vi "ALTS-2015 Write Robot on OPC.vi"(7 "Option":T1=enum."Write Invalid Serial Task", 8 "error in (no error)":errorcluster, 10 "Station # Load":T2, 11 "Serial Details in":T3) -> (0 "error out":errorcluster)   [LabVIEW 2013]
uses:
  Controls/ALTS-2015 Serial Details.ctl
  Controls/ALTS-2015 Station Cluster.ctl
  Controls/ALTS-2015 Write Robot Task OPC Options.ctl
  OPC Engine/Controls/ALTS-2015 OPC Write Global Options.ctl
  OPC Engine/Controls/ALTS-2015 OPC Write Registers.ctl
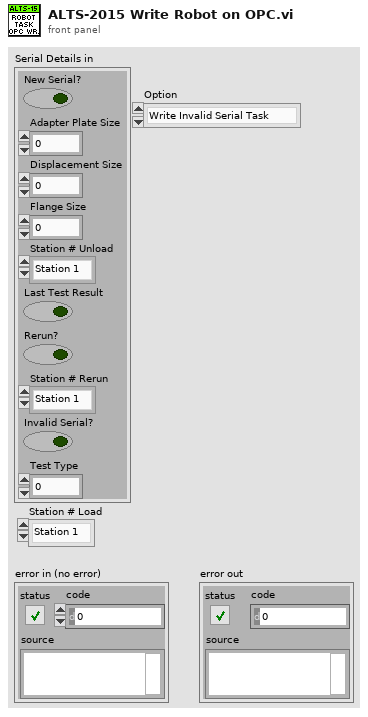
[diagram p1: front panel]
types:
  T1 = typedef "ALTS-2015 Write Robot Task OPC Options.ctl" = enum16{"Write New Serial Task", "Write Rerun Task", "Write Unload Task", "Write Invalid Serial Task"}
  T2 = typedef "ALTS-2015 Station Cluster.ctl" = enum16{"Station 1", "Station 2", "Station 3", "Station 4"}
  T3 = typedef "ALTS-2015 Serial Details.ctl" = cluster{"New Serial?":bool, "Adapter Plate Size":i32, "Displacement Size":i32, "Flange Size":i32, "Station # Unload":T2, "Last Test Result":bool, "Rerun?":bool, "Station # Rerun":T2, "Invalid Serial?":bool, "Test Type":i32}
  T4 = typedef "ALTS-2015 OPC Write Global Options.ctl" = enum16{"Init", "Write Value", "Write Array", "Read Value", "Read Array", "Read All"}
  T5 = typedef "ALTS-2015 OPC Write Registers.ctl" = enum16{"Task Ready for Robot", "New Part", "Serial Adapter Size", "Serial Displacement Size", "Serial Flange Size", "Last Test Result", "Station Number", "Rerun", "Invalid SNo", "PC ACK Read Tags"}
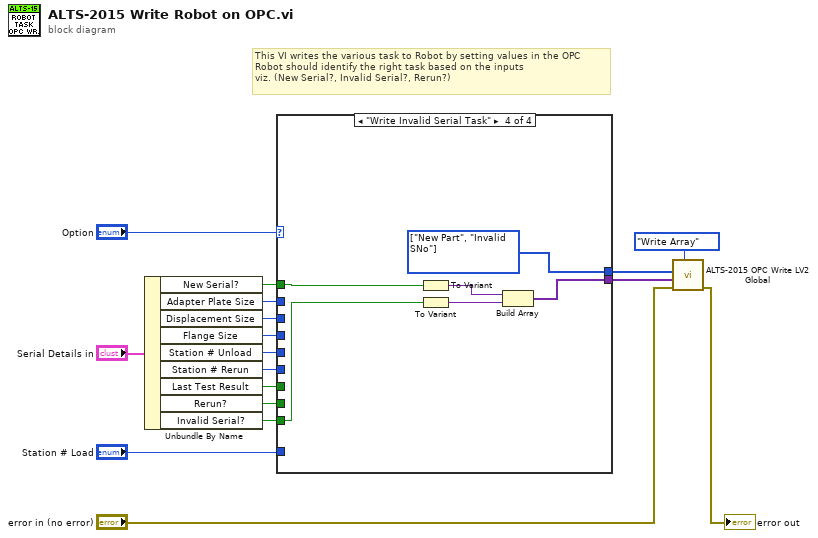
[diagram p0: block diagram]
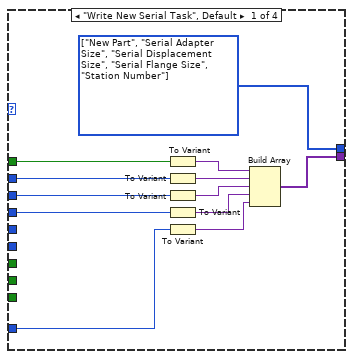
[diagram p2: hidden frame]
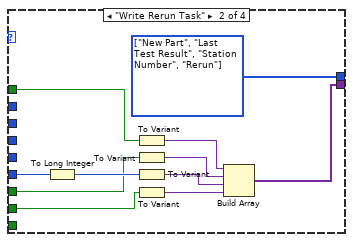
[diagram p3: hidden frame]
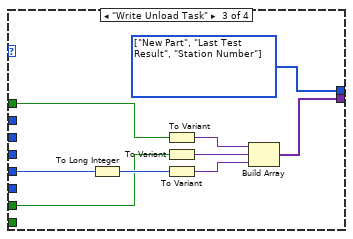
[diagram p4: hidden frame]
diagram:
  # "This VI writes the various task to Robot by setting values in the OPC\nRobot should identify the right task based on the inputs \nviz. (New Serial?, Invalid Serial?, Rerun?)"
  n1 = Unbundle By Name("Serial Details in") -> ("New Serial?"=w11:bool, "Adapter Plate Size"=w12:i32, "Displacement Size"=w13:i32, "Flange Size"=w16:i32, "Station # Unload"=w3:T2, "Station # Rerun"=w4:T2, "Last Test Result"=w5:bool, "Rerun?"=w2:bool, "Invalid Serial?"=w6:bool)
  n2 = case shown="\"Write Invalid Serial Task\"" "Option" {
    tunnel: [w29 w34 w45 w52] -> w17
    tunnel: w16 -> [w28 _ _ _]
    tunnel: [w27 w35 w44 w53] -> w15
    tunnel: w13 -> [w26 _ _ _]
    tunnel: w12 -> [w25 _ _ _]
    tunnel: w11 -> [w24 w33 w43 w51]
    tunnel: w6 -> [_ _ _ w50]
    tunnel: w5 -> [_ w32 w42 _]
    tunnel: w4 -> [_ w31 _ _]
    tunnel: w3 -> [_ _ w41 _]
    tunnel: w2 -> [_ w30 _ _]
    tunnel: "Station # Load" -> [w18 _ _ _]
    frame "Write New Serial Task", Default {
      w27 = T5[] [enum."New Part", enum."Serial Adapter Size", enum."Serial Displacement Size", enum."Serial Flange Size", enum."Station Number"] items=["Task Ready for Robot", "New Part", "Serial Adapter Size", "Serial Displacement Size", "Serial Flange Size", "Last Test Result", "Station Number", "Rerun", "Invalid SNo", "PC ACK Read Tags"] ("OPC Write Register Array")
      n3 = To Variant(anything=w24) -> (Variant=w23:variant)
      n4 = To Variant(anything=w25) -> (Variant=w22:variant)
      n5 = To Variant(anything=w26) -> (Variant=w21:variant)
      n6 = To Variant(anything=w28) -> (Variant=w20:variant)
      n7 = To Variant(anything=w18) -> (Variant=w19:variant)
      n8 = Build Array(w23, w22, w21, w20, w19) -> (w29:variant[])
    }
    frame "Write Rerun Task" {
      w35 = T5[] [enum."New Part", enum."Last Test Result", enum."Station Number", enum."Rerun"] items=["Task Ready for Robot", "New Part", "Serial Adapter Size", "Serial Displacement Size", "Serial Flange Size", "Last Test Result", "Station Number", "Rerun", "Invalid SNo", "PC ACK Read Tags"] ("OPC Write Register Array")
      n9 = To Long Integer(number=w31) -> (32bit integer=w36:i32)
      n10 = To Variant(anything=w33) -> (Variant=w40:variant)
      n11 = To Variant(anything=w32) -> (Variant=w39:variant)
      n12 = To Variant(anything=w36) -> (Variant=w38:variant)
      n13 = To Variant(anything=w30) -> (Variant=w37:variant)
      n14 = Build Array(w40, w39, w38, w37) -> (w34:variant[])
    }
    frame "Write Unload Task" {
      w44 = T5[] [enum."New Part", enum."Last Test Result", enum."Station Number"] items=["Task Ready for Robot", "New Part", "Serial Adapter Size", "Serial Displacement Size", "Serial Flange Size", "Last Test Result", "Station Number", "Rerun", "Invalid SNo", "PC ACK Read Tags"] ("OPC Write Register Array")
      n15 = To Long Integer(number=w41) -> (32bit integer=w46:i32)
      n16 = To Variant(anything=w43) -> (Variant=w49:variant)
      n17 = To Variant(anything=w42) -> (Variant=w48:variant)
      n18 = To Variant(anything=w46) -> (Variant=w47:variant)
      n19 = Build Array(w49, w48, w47) -> (w45:variant[])
    }
    frame "Write Invalid Serial Task" {
      w53 = T5[] [enum."New Part", enum."Invalid SNo"] items=["Task Ready for Robot", "New Part", "Serial Adapter Size", "Serial Displacement Size", "Serial Flange Size", "Last Test Result", "Station Number", "Rerun", "Invalid SNo", "PC ACK Read Tags"] ("OPC Write Register Array")
      n20 = To Variant(anything=w51) -> (Variant=w55:variant)
      n21 = To Variant(anything=w50) -> (Variant=w54:variant)
      n22 = Build Array(w55, w54) -> (w52:variant[])
    }
  }
  n23 = call "ALTS-2015 OPC Write LV2 Global.vi"("Options"=ALTS-2015_OPC_Write_Global_Options."Write Array", "error in (no error)"="error in (no error)", "OPC value"=w17, "OPC Write Register Array"=w15) -> ("error out"=→"error out":errorcluster)  [unwired: 5 in, 2 out]
